vi "STS_zOffset.vi"() -> ()   [LabVIEW 2014]
uses:
  <userlib>/Nanonis Prog Interface V5/Nanonis Prog Interface.lvlib
panel:
  out "Z position (m)":sgl format="%#_6p"
  in  "STS z offset":dbl=-1.7e-10 format="%#_6p"
  in  "STS Bias":dbl=0.1 format="%#_6p"
  in  "STS Current":dbl=1e-10 format="%#_6p"
  in  "preSTS delay [ms]":u32=1000
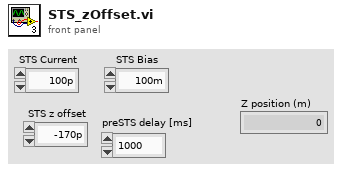
[diagram p1: front panel]
types:
  T1 = cluster{"Z-Controller Hold":bool, "Record final Z":bool, "Reset Bias":bool}
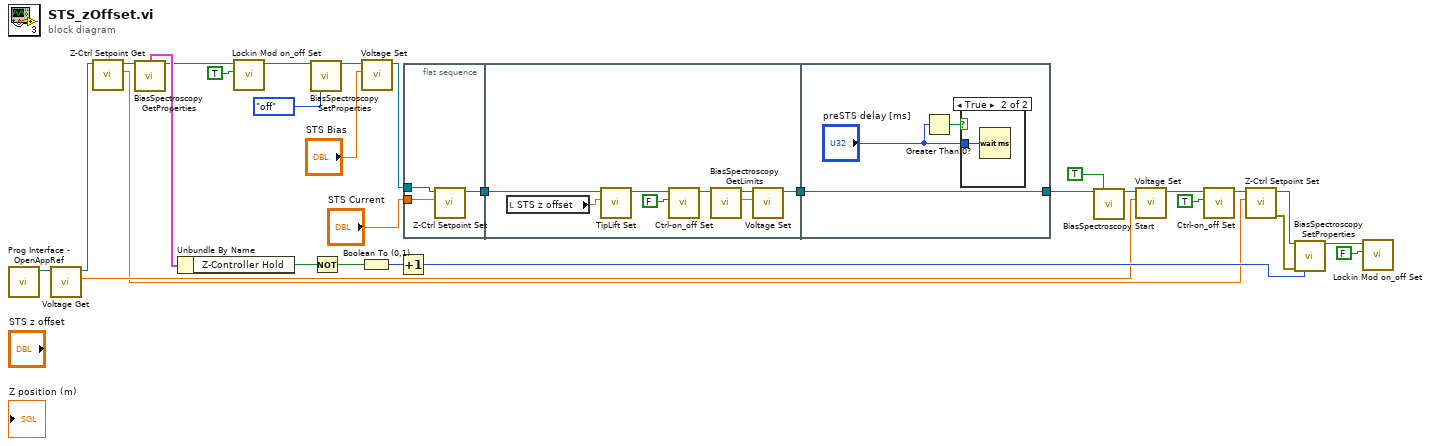
[diagram p0: block diagram]
diagram:
  n1 = call <userlib>:"Prog Interface - OpenAppRef.vi"() -> ("Application reference"=w5:refnum<vi>)  [unwired: 6 in, 1 out]
  n2 = call <userlib>:"Voltage Get.vi"("Application ref in"=w5) -> ("Bias (V)"=w2:sgl, "Application ref out"=w4:refnum<vi>)  [unwired: 8 in, 1 out]
  n3 = call <userlib>:"Z-Ctrl Setpoint Get.vi"("Application ref in"=w4) -> ("Z Controller setpoint"=w1:sgl, "Application ref out"=w3:refnum<vi>)  [unwired: 7 in, 1 out]
  n4 = call <userlib>:"BiasSpectroscopy GetProperties.vi"("Application ref in"=w3) -> ("Advanced options"=w19:T1, "Application ref out"=w12:refnum<vi>)  [unwired: 6 in, 7 out]
  n5 = Unbundle By Name(w19) -> ("Z-Controller Hold"=w18:bool)
  n6 = call <userlib>:"Lockin Mod on_off Set.vi"("Lockin ON/OFF"=TRUE, "Application ref in"=w12) -> ("Application ref out"=w11:refnum<vi>)  [unwired: 8 in, 1 out]
  n7 = call <userlib>:"BiasSpectroscopy SetProperties.vi"("Application ref in"=w11, "Z-Controller hold (no change)"=enum16{"no change", "on", "off"}."off") -> ("Application ref out"=w14:refnum<vi>)  [unwired: 12 in, 1 out]
  n8 = Not(x=w18) -> (.not. x?=w15:bool)
  n9 = Boolean To (0,1)(Boolean=w15) -> (0, 1=w17:i16)
  n10 = call <userlib>:"Voltage Set.vi"("Bias (V)"="STS Bias", "Application ref in"=w14) -> ("Application ref out"=w28:refnum<vi>)  [unwired: 8 in, 1 out]
  n11 = Increment(x=w17) -> (x+1=w16:i16)
  n12 = flat-sequence {
    tunnel: w28 -> [w33]
    tunnel: "STS Current" -> [w31]
    tunnel: [w32] -> w30
    tunnel: w30 -> [w35]
    tunnel: [w37] -> w13
    tunnel: [w44] -> w27
    tunnel: w13 -> [w44]
    frame #0 {
      n13 = call <userlib>:"Z-Ctrl Setpoint Set.vi"("Z Controller setpoint"=w31, "Application ref in"=w33) -> ("Application ref out"=w32:refnum<vi>)  [unwired: 8 in, 1 out]
    }
    frame #1 {
      n14 = local read "STS z offset"() -> (w36:dbl)
      n15 = call <userlib>:"TipLift Set.vi"("TipLift (m)"=w36, "Application ref in"=w35) -> ("Application ref out"=w34:refnum<vi>)  [unwired: 8 in, 1 out]
      n16 = call <userlib>:"Ctrl-on_off Set.vi"("Z Controller ON/OFF"=FALSE, "Application ref in"=w34) -> ("Application ref out"=w39:refnum<vi>)  [unwired: 8 in, 1 out]
      n17 = call <userlib>:"BiasSpectroscopy GetLimits.vi"("Application ref in"=w39) -> ("Start value (V)"=w38:sgl, "Application ref out"=w40:refnum<vi>)  [unwired: 5 in, 2 out]
      n18 = call <userlib>:"Voltage Set.vi"("Bias (V)"=w38, "Application ref in"=w40) -> ("Application ref out"=w37:refnum<vi>)  [unwired: 8 in, 1 out]
    }
    frame #2 {
      n19 = Greater Than 0?(x="preSTS delay [ms]") -> (x > 0?=w42:bool)
      n20 = case shown="True" w42 {
        tunnel: "preSTS delay [ms]" -> [_ w45]
        frame False {
        }
        frame True {
          n21 = Wait (ms)(milliseconds to wait=w45) -> ()  [unwired: 1 out]
        }
      }
    }
  }
  n22 = call <userlib>:"BiasSpectroscopy Start.vi"("Application ref in"=w27, "Get data (F)"=TRUE ("Get Data (F)")) -> ("Application ref out"=w23:refnum<vi>)  [unwired: 9 in, 4 out]
  n23 = call <userlib>:"Voltage Set.vi"("Bias (V)"=w2, "Application ref in"=w23) -> ("Application ref out"=w25:refnum<vi>)  [unwired: 8 in, 1 out]
  n24 = call <userlib>:"Ctrl-on_off Set.vi"("Z Controller ON/OFF"=TRUE, "Application ref in"=w25) -> ("Application ref out"=w24:refnum<vi>)  [unwired: 8 in, 1 out]
  n25 = call <userlib>:"Z-Ctrl Setpoint Set.vi"("Z Controller setpoint"=w1, "Application ref in"=w24) -> ("error out"=w20:errorcluster, "Application ref out"=w21:refnum<vi>)  [unwired: 8 in]
  n26 = call <userlib>:"BiasSpectroscopy SetProperties.vi"("Application ref in"=w21, "Error in (no error)"=w20, "Z-Controller hold (no change)"=w16) -> ("Application ref out"=w9:refnum<vi>)  [unwired: 11 in, 1 out]
  n27 = call <userlib>:"Lockin Mod on_off Set.vi"("Lockin ON/OFF"=FALSE, "Application ref in"=w9) -> ()  [unwired: 8 in, 2 out]
